vi "Read Swerve Encoders.vi"(1 "BL Ref":T1={"DevStatus"={"status"=FALSE, "code"=0, "source"=""}, "Analog Channel"=enum."Invalid"}, 2 "BR Ref":T1={"DevStatus"={"status"=FALSE, "code"=0, "source"=""}, "Analog Channel"=enum."Invalid"}, 3 "FL Ref":T1={"DevStatus"={"status"=FALSE, "code"=0, "source"=""}, "Analog Channel"=enum."Invalid"}, 4 "FR Ref":T1={"DevStatus"={"status"=FALSE, "code"=0, "source"=""}, "Analog Channel"=enum."Invalid"}) -> ()   [LabVIEW 2020]
uses:
  <vilib>/Rock Robotics/WPI/AnalogChannel/WPI_AnalogChannelDevRef.ctl
  <vilib>/Rock Robotics/SystemInterfaces/AI/FPGA_AIChannel.ctl
  Robot Global Data.vi
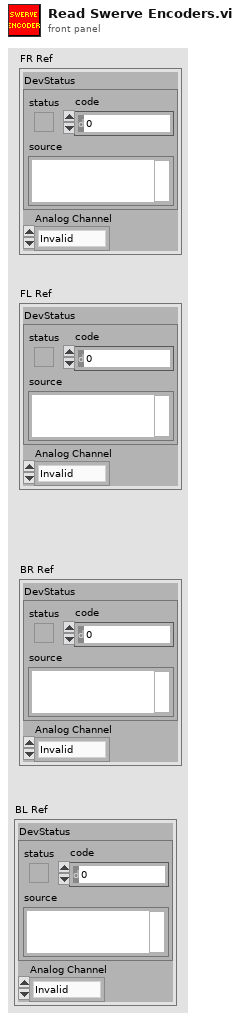
[diagram p1: front panel]
types:
  T1 = typedef "WPI_AnalogChannelDevRef.ctl" = cluster{"DevStatus":errorcluster, "Analog Channel":T2}
  T2 = typedef "FPGA_AIChannel.ctl" = enum8{"AI 0", "AI 1", "AI 2", "AI 3", "AI MXP 0", "AI MXP 1", "AI MXP 2", "AI MXP 3", "Invalid"}
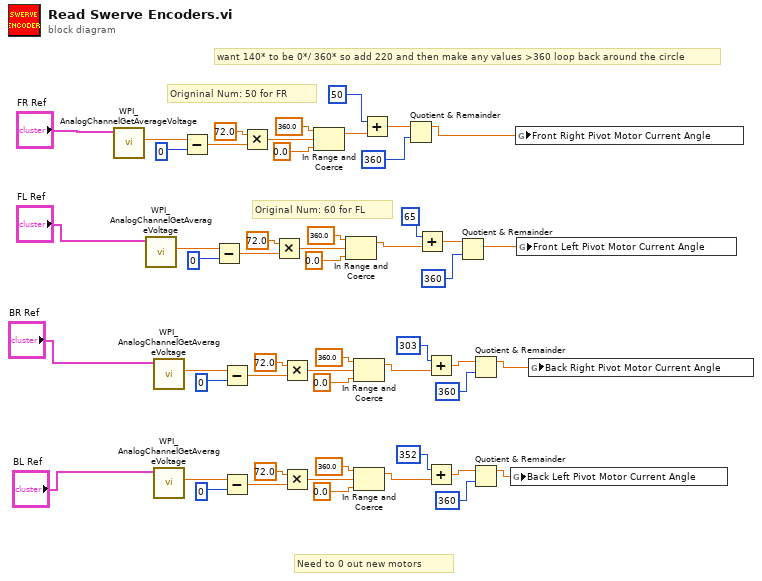
[diagram p0: block diagram]
diagram:
  # "Original Num: 60 for FL"
  # "Origninal Num: 50 for FR"
  # "Need to 0 out new motors"
  # "want 140* to be 0*/ 360* so add 220 and then make any values >360 loop back around the circle"
  n1 = call <vilib>:"WPI_AnalogChannelGetAverageVoltage.vi"("AIDeviceRef"="FR Ref") -> ("Voltage"=w49:dbl)  [unwired: 1 in, 9 out]
  n2 = call <vilib>:"WPI_AnalogChannelGetAverageVoltage.vi"("AIDeviceRef"="FL Ref") -> ("Voltage"=w42:dbl)  [unwired: 1 in, 9 out]
  n3 = call <vilib>:"WPI_AnalogChannelGetAverageVoltage.vi"("AIDeviceRef"="BR Ref") -> ("Voltage"=w35:dbl)  [unwired: 1 in, 9 out]
  n4 = call <vilib>:"WPI_AnalogChannelGetAverageVoltage.vi"("AIDeviceRef"="BL Ref") -> ("Voltage"=w10:dbl)  [unwired: 1 in, 9 out]
  n5 = Subtract(x=w49, y=0) -> (x-y=w52:dbl)
  n6 = Subtract(x=w42, y=0) -> (x-y=w45:dbl)
  n7 = Subtract(x=w35, y=0) -> (x-y=w38:dbl)
  n8 = Subtract(x=w10, y=0) -> (x-y=w13:dbl)
  n9 = Multiply(x=72.0, y=w52) -> (x*y=w46:dbl)
  n10 = Multiply(x=72.0, y=w45) -> (x*y=w39:dbl)
  n11 = Multiply(x=72.0, y=w38) -> (x*y=w32:dbl)
  n12 = Multiply(x=72.0, y=w13) -> (x*y=w7:dbl)
  n13 = In Range and Coerce(upper limit=360.0, x=w46, lower limit=0.0 ("upper limit")) -> (coerced(x)=w28:dbl)  [unwired: 1 out]
  n14 = In Range and Coerce(upper limit=360.0, x=w39, lower limit=0.0 ("upper limit")) -> (coerced(x)=w18:dbl)  [unwired: 1 out]
  n15 = In Range and Coerce(upper limit=360.0, x=w32, lower limit=0.0 ("upper limit")) -> (coerced(x)=w23:dbl)  [unwired: 1 out]
  n16 = In Range and Coerce(upper limit=360.0, x=w7, lower limit=0.0 ("upper limit")) -> (coerced(x)=w6:dbl)  [unwired: 1 out]
  n17 = Add(x=50, y=w28) -> (x+y=w26:dbl)
  n18 = Quotient & Remainder(x=w26, y=360) -> (x-y*floor(x/y)=w24:dbl)  [unwired: 1 out]
  n19 = Add(x=65, y=w18) -> (x+y=w16:dbl)
  n20 = Add(x=303, y=w23) -> (x+y=w21:dbl)
  n21 = Add(x=352, y=w6) -> (x+y=w4:dbl)
  n22 = Quotient & Remainder(x=w16, y=360) -> (x-y*floor(x/y)=w15:dbl)  [unwired: 1 out]
  n23 = Quotient & Remainder(x=w21, y=360) -> (x-y*floor(x/y)=w20:dbl)  [unwired: 1 out]
  n24 = Quotient & Remainder(x=w4, y=360) -> (x-y*floor(x/y)=w3:dbl)  [unwired: 1 out]
  n25 = global write "Robot Global Data.vi" "Back Left Pivot Motor Current Angle"(w3) -> ()
  n26 = global write "Robot Global Data.vi" "Front Right Pivot Motor Current Angle"(w24) -> ()
  n27 = global write "Robot Global Data.vi" "Front Left Pivot Motor Current Angle"(w15) -> ()
  n28 = global write "Robot Global Data.vi" "Back Right Pivot Motor Current Angle"(w20) -> ()
